vi "PV HLT5xx Start calibrate.vi"(7 "Adress of unit":u16=1 min=1 max=999 step=1, 8 "error in (no error)":errorcluster, 11 "VISA session":refnum<visa-resource-name>) -> (0 "error out":errorcluster, 2 "response (data)":string, 3 "dup VISA session":refnum<visa-resource-name>)   [LabVIEW 2016, in "Pfeiffer Vacuum.lvlib"]
doc: "This VI allows you to set or check the \"Start Calibration (Para 699)\" on the SmartTest (HLT5xx)."
uses:
  Pfeiffer Vacuum.lvlib
panel:
  # "Start Calibration"
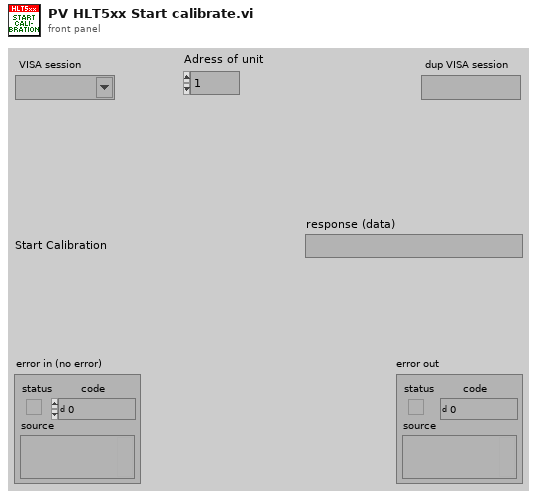
[diagram p1: front panel]
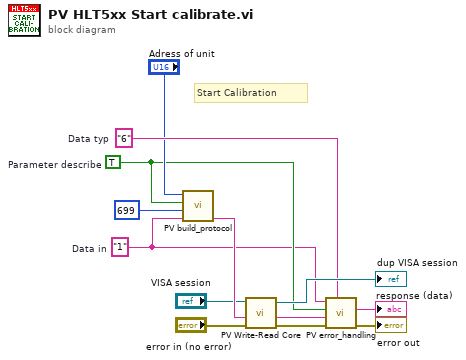
[diagram p0: block diagram]
diagram:
  w1 = "1"  # Data in
  w2 = TRUE  # Parameter describe
  w8 = "6"  # Data typ
  # "Start Calibration"
  n1 = call "PV build_protocol.vi"("Data"=w1, "Parameter-number"=u16 699, "parameter\nread<->describe"=w2, "Adress"="Adress of unit") -> ("output"=w12:string)  [unwired: 3 in]
  n2 = call "PV Write-Read Core.vi"("error in"="error in (no error)", "Write data in"=w12, "VISA session"="VISA session") -> ("error out"=w10:errorcluster, "response (data) out"=w11:string, "dup VISA session"=→"dup VISA session":refnum<visa-resource-name>)  [unwired: 2 in]
  n3 = call "PV error_handling.vi"("Data Typ in"=w8, "error in"=w10, "response (data) in"=w11, "Parameter\nread only<->describe"=w2, "data in"=w1) -> ("error out"=→"error out":errorcluster, "Data out"=→"response (data)":string)  [unwired: 4 in, 1 out]
